vi "Hindbrain.vi"() -> ()   [LabVIEW 2010]
doc: "Hindbrain_RobotBrainExample. This VI is an example of the Hindbrain layer of the Olin Robot Architecture. It collects all SENSE data and sends it up three neural clusters to the Midbrain and accepts one ACT cluster from Midbrain to drive all robot actuators."
uses:
  GlobalWhatAroundMe.vi
  GlobalWhereAmI.vi
  GlobalACT.vi
  GlobalHowAmI.vi
panel:
  out "WhereSensor":T1
  out "Act Command":cluster{"Velocity":dbl, "Direction":dbl}
  out "Act":bool
  out "How?":bool
  out "What?":bool
  in  "stop":bool
  out "Where":bool
  out "HowAmI?":cluster{"T":dbl, "Battery":dbl, "Temp":dbl}
  out "WhatAroundMe?":cluster{"T":dbl, "Range":dbl, "Bearing":dbl}[](array[cluster])
  # "must un-stop for new run"
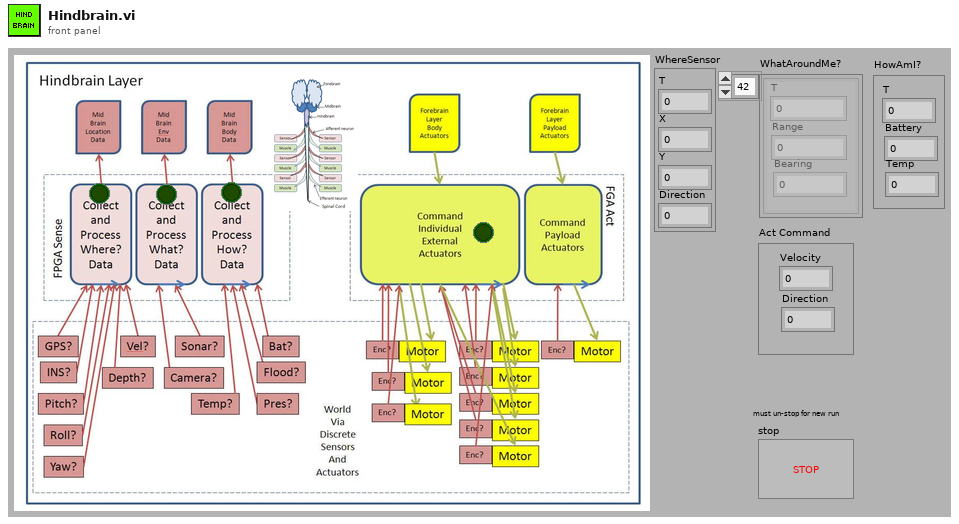
[diagram p1: front panel]
types:
  T1 = cluster{"T":dbl, "X":dbl, "Y":dbl, "Direction":dbl}
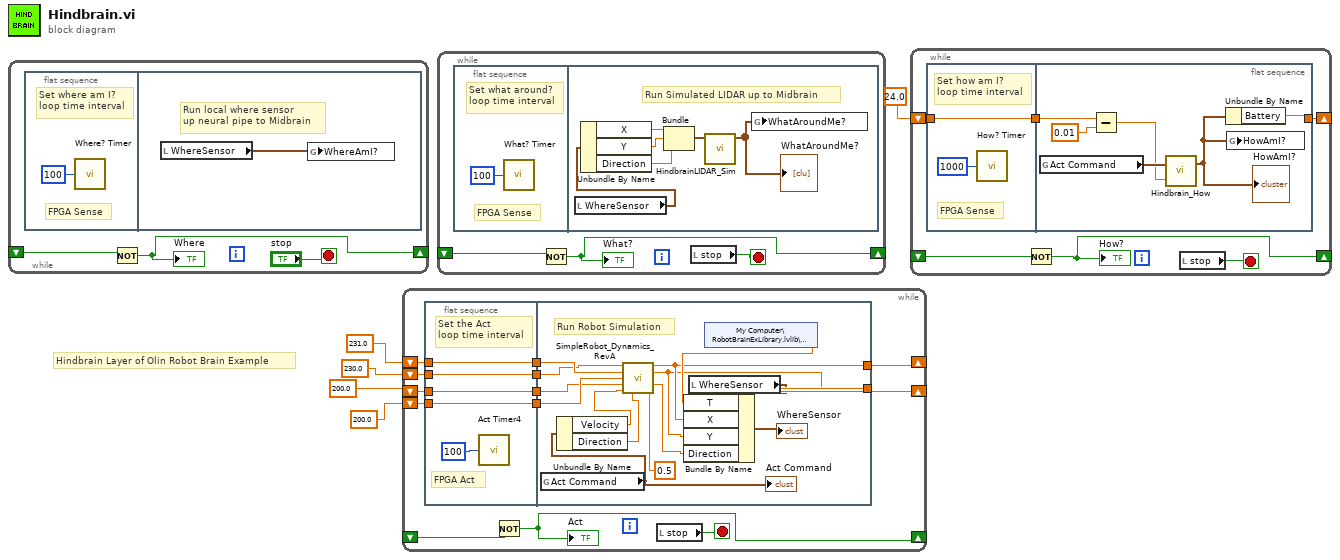
[diagram p0: block diagram]
diagram:
  # "Hindbrain Layer of Olin Robot Brain Example"
  n1 = while {
    shift-right: [w6] -> _
    shift-left: _ -> [w7]
    stop <- "stop" stop-if-true
    n2 = flat-sequence {
      frame #0 {
        # "FPGA Sense"
        # "Set where am I?\nloop time interval"
        n3 = call "Where? Timer"("Count(mSec)"=u32 100) -> ()  [unwired: 1 out]
      }
      frame #1 {
        # "Run local where sensor\nup neural pipe to Midbrain"
        n4 = local read "WhereSensor"() -> (w10:T1)
        n5 = global write "GlobalWhereAmI.vi" "WhereAmI?"(w10) -> ()
      }
    }
    n6 = Not(x=w7) -> (.not. x?=w6:bool)
    "Where" <- w6
  }
  n7 = while {
    shift-right: [w22] -> _
    shift-left: _ -> [w23]
    shift-right: [w18] -> _
    shift-left: 231.0 ("x 2") -> [w19]
    shift-left: 230.0 ("x 2") -> [w16]
    shift-right: [w13] -> _
    shift-left: 200.0 ("y 2") -> [w14]
    shift-left: 200.0 ("y 2") -> [w11]
    stop <- w21 stop-if-true
    n8 = flat-sequence {
      tunnel: [w27] -> w20
      tunnel: w19 -> [w27]
      tunnel: [w26] -> w17
      tunnel: w16 -> [w26]
      tunnel: [w25] -> w15
      tunnel: w14 -> [w25]
      tunnel: [w24] -> w12
      tunnel: w11 -> [w24]
      tunnel: w20 -> [w32]
      tunnel: [w37] -> w18
      tunnel: w17 -> [w31]
      tunnel: w15 -> [w29]
      tunnel: [w36] -> w13
      tunnel: w12 -> [w30]
      frame #0 {
        # "FPGA Act"
        # "Set the Act\nloop time interval"
        n9 = call "Act Timer4"("Count(mSec)"=u32 100) -> ()  [unwired: 1 out]
      }
      frame #1 {
        # "Run Robot Simulation"
        n10 = global read "GlobalACT.vi" "Act Command"() -> (w42:cluster{"Velocity":dbl, "Direction":dbl})
        "Act Command" <- w42
        n11 = Unbundle By Name(w42) -> ("Velocity"=w41:dbl, "Direction"=w40:dbl)
        n12 = call "SimpleRobot_Dynamics_RevA.vi"("x0"=w31, "x1"=w32, "y0"=w30, "y1"=w29, "Velocity"=w41, "Direction"=w40, "DeltaT (timestep)"=0.5) -> ("x 2"=w37:dbl, "y 2"=w36:dbl, "Direction 2"=w35:dbl)  [unwired: 6 in]
        n13 = local read "WhereSensor"() -> (w33:T1)
        n14 = shared-variable "My Computer\\RobotBrainExLibrary.lvlib\\MissionTime"() -> (w38:dbl)  [unwired: 1 in, 1 out]
        n15 = Bundle By Name(cluster=w33, "T"=w38, "X"=w37, "Y"=w36, "Direction"=w35) -> (→"WhereSensor":T1)
      }
    }
    n16 = Not(x=w23) -> (.not. x?=w22:bool)
    "Act" <- w22
    n17 = local read "stop"() -> (w21:bool)
  }
  n18 = while {
    shift-right: [w44] -> _
    shift-left: _ -> [w45]
    stop <- w43 stop-if-true
    n19 = flat-sequence {
      frame #0 {
        # "FPGA Sense"
        # "Set what around?\nloop time interval"
        n20 = call "What? Timer"("Count(mSec)"=u32 100) -> ()  [unwired: 1 out]
      }
      frame #1 {
        # "Run Simulated LIDAR up to Midbrain"
        n21 = local read "WhereSensor"() -> (w51:T1)
        n22 = Unbundle By Name(w51) -> ("X"=w49:dbl, "Y"=w48:dbl, "Direction"=w47:dbl)
        n23 = Bundle("X"=w49, "Y"=w48, "Direction"=w47) -> (w50:cluster{"X":dbl, "Y":dbl, "Direction":dbl})  [unwired: 1 in]
        n24 = call "HindbrainLIDAR_Sim.vi"("SubPosition"=w50) -> ("WhatAroundMe?"=w52:cluster{"T":dbl, "Range":dbl, "Bearing":dbl}[])  [unwired: 10 in]
        "WhatAroundMe?" <- w52
        n25 = global write "GlobalWhatAroundMe.vi" "WhatAroundMe?"(w52) -> ()
      }
    }
    n26 = Not(x=w45) -> (.not. x?=w44:bool)
    "What?" <- w44
    n27 = local read "stop"() -> (w43:bool)
  }
  n28 = while {
    shift-right: [w57] -> _
    shift-left: _ -> [w58]
    shift-right: [w53] -> _
    shift-left: 24.0 -> [w54]
    stop <- w56 stop-if-true
    n29 = flat-sequence {
      tunnel: [w59] -> w55
      tunnel: w54 -> [w59]
      tunnel: w55 -> [w65]
      tunnel: [w61] -> w53
      frame #0 {
        # "FPGA Sense"
        # "Set how am I?\nloop time interval"
        n30 = call "How? Timer"("Count(mSec)"=u32 1000) -> ()  [unwired: 1 out]
      }
      frame #1 {
        n31 = global read "GlobalACT.vi" "Act Command"() -> (w64:cluster{"Velocity":dbl, "Direction":dbl})
        n32 = Subtract(x=w65, y=0.01) -> (x-y=w63:dbl)
        n33 = call "Hindbrain_How.vi"("Battery"=w63, "Act Command"=w64) -> ("HowAmI?"=w62:cluster{"T":dbl, "Battery":dbl, "Temp":dbl})  [unwired: 1 in]
        "HowAmI?" <- w62
        n34 = Unbundle By Name(w62) -> ("Battery"=w61:dbl)
        n35 = global write "GlobalHowAmI.vi" "HowAmI?"(w62) -> ()
      }
    }
    n36 = Not(x=w58) -> (.not. x?=w57:bool)
    "How?" <- w57
    n37 = local read "stop"() -> (w56:bool)
  }
